vi "Restarts by Flow Sandbox Original.vi"() -> ()   [LabVIEW 2013]
uses:
  Type Defs/CAN Mode.ctl
  Type Defs/Controller Names.ctl
  Type Defs/Controller List.ctl
  <vilib>/FPGAPlugInAG/sbRIO-9626/niLvFpga_Open_sbRIO-9626.vi
  <vilib>/rvi/interface/common/dynamic/niFpgaDynamicAddResources.vi
  <vilib>/rvi/interface/common/niFpgaWaitOnOcc.vi
  <vilib>/Utility/error.llb/Error Cluster From Error Code.vi
  <vilib>/rvi/errors/niLvFpgaAdjustHostInterfaceError.vi
  <vilib>/FPGAPlugInAG/Dynamic/niLvFpga_Reset_Dynamic.vi
  <vilib>/FPGAPlugInAG/Dynamic/niLvFpga_Run_Dynamic.vi
  <vilib>/rvi/interface/nirviOpenFPGA/nirviOpenFPGA.xnode
  FPGA/bitfiles/RestartsbyFlowOriginal.lvbitx
  <vilib>/rvi/interface/nirviMethod/nirviMethod.xnode
  <vilib>/rvi/interface/nirviReadWriteControl/nirviReadWriteControl.xnode
  NiFpgaLv.dll
  <vilib>/rvi/interface/Simulation/niFpgaSimulationCallBeginRW.vi
  <vilib>/NI_Real-Time Target Support.lvlib
  <vilib>/FPGAPlugInAG/Dynamic/niLvFpga_ReadFifo_Dynamic.vi
  <vilib>/rvi/errors/niLvFpgaMergeErrorWithErrorCode.vi
  <vilib>/FPGAPlugInAG/Dynamic/niLvFpga_ConfigureFifo_Dynamic.vi
panel:
  out "Pressure":dbl
  out "DetPres Starts":u32
  out "Pressure Graph":dbl[][](graph)
  out "Reset Restarts 2":bool
  out "Negative Threshold":dbl
  out "Positive Threshold":dbl
  out "Armed":bool
  out "Flow":dbl
  out "Alt Flow Starts":u32
  out "Current":fxp<+/-,28,17>
  out "Current Graph":dbl[](graph)
  out "Init 2 Index":i32
  out "Commanded Starts":i16
  in  "Update Graph":bool=TRUE
  out "DetFlow Starts":u32
  in  "Position":i32=1
  in  "Seconds per Step":dbl=1.5 min=0.25 max=500.0 step=0.25
  out "Case":string
  in  "PreDataPts":i32=2000
  in  "Stop Init 2":bool
  out "Data Points":u32
  out "Current Step":i32
  in  "Reset Restarts":bool
  out "Flow Graph":dbl[](graph)
  in  "Profile":dbl[][](array[numeric])=[[1.25, 0.0, 0.0], [1.25, 650.0, 700.0]]
  in  "Run profile?":bool
  out "CFR 2":u64 format="%.0x"
  out "CFR2":u64 format="%.0x"
  in  "Pressure":dbl min=0.0 max=800.0 step=1.0 format="%#_13g"
  out "CPU Usage:":dbl=7.74131899555212 format="%.1f"
  in  "CAN CMD":dbl min=0.0 max=800.0 step=1.0
  # "cmd"
  # "pres"
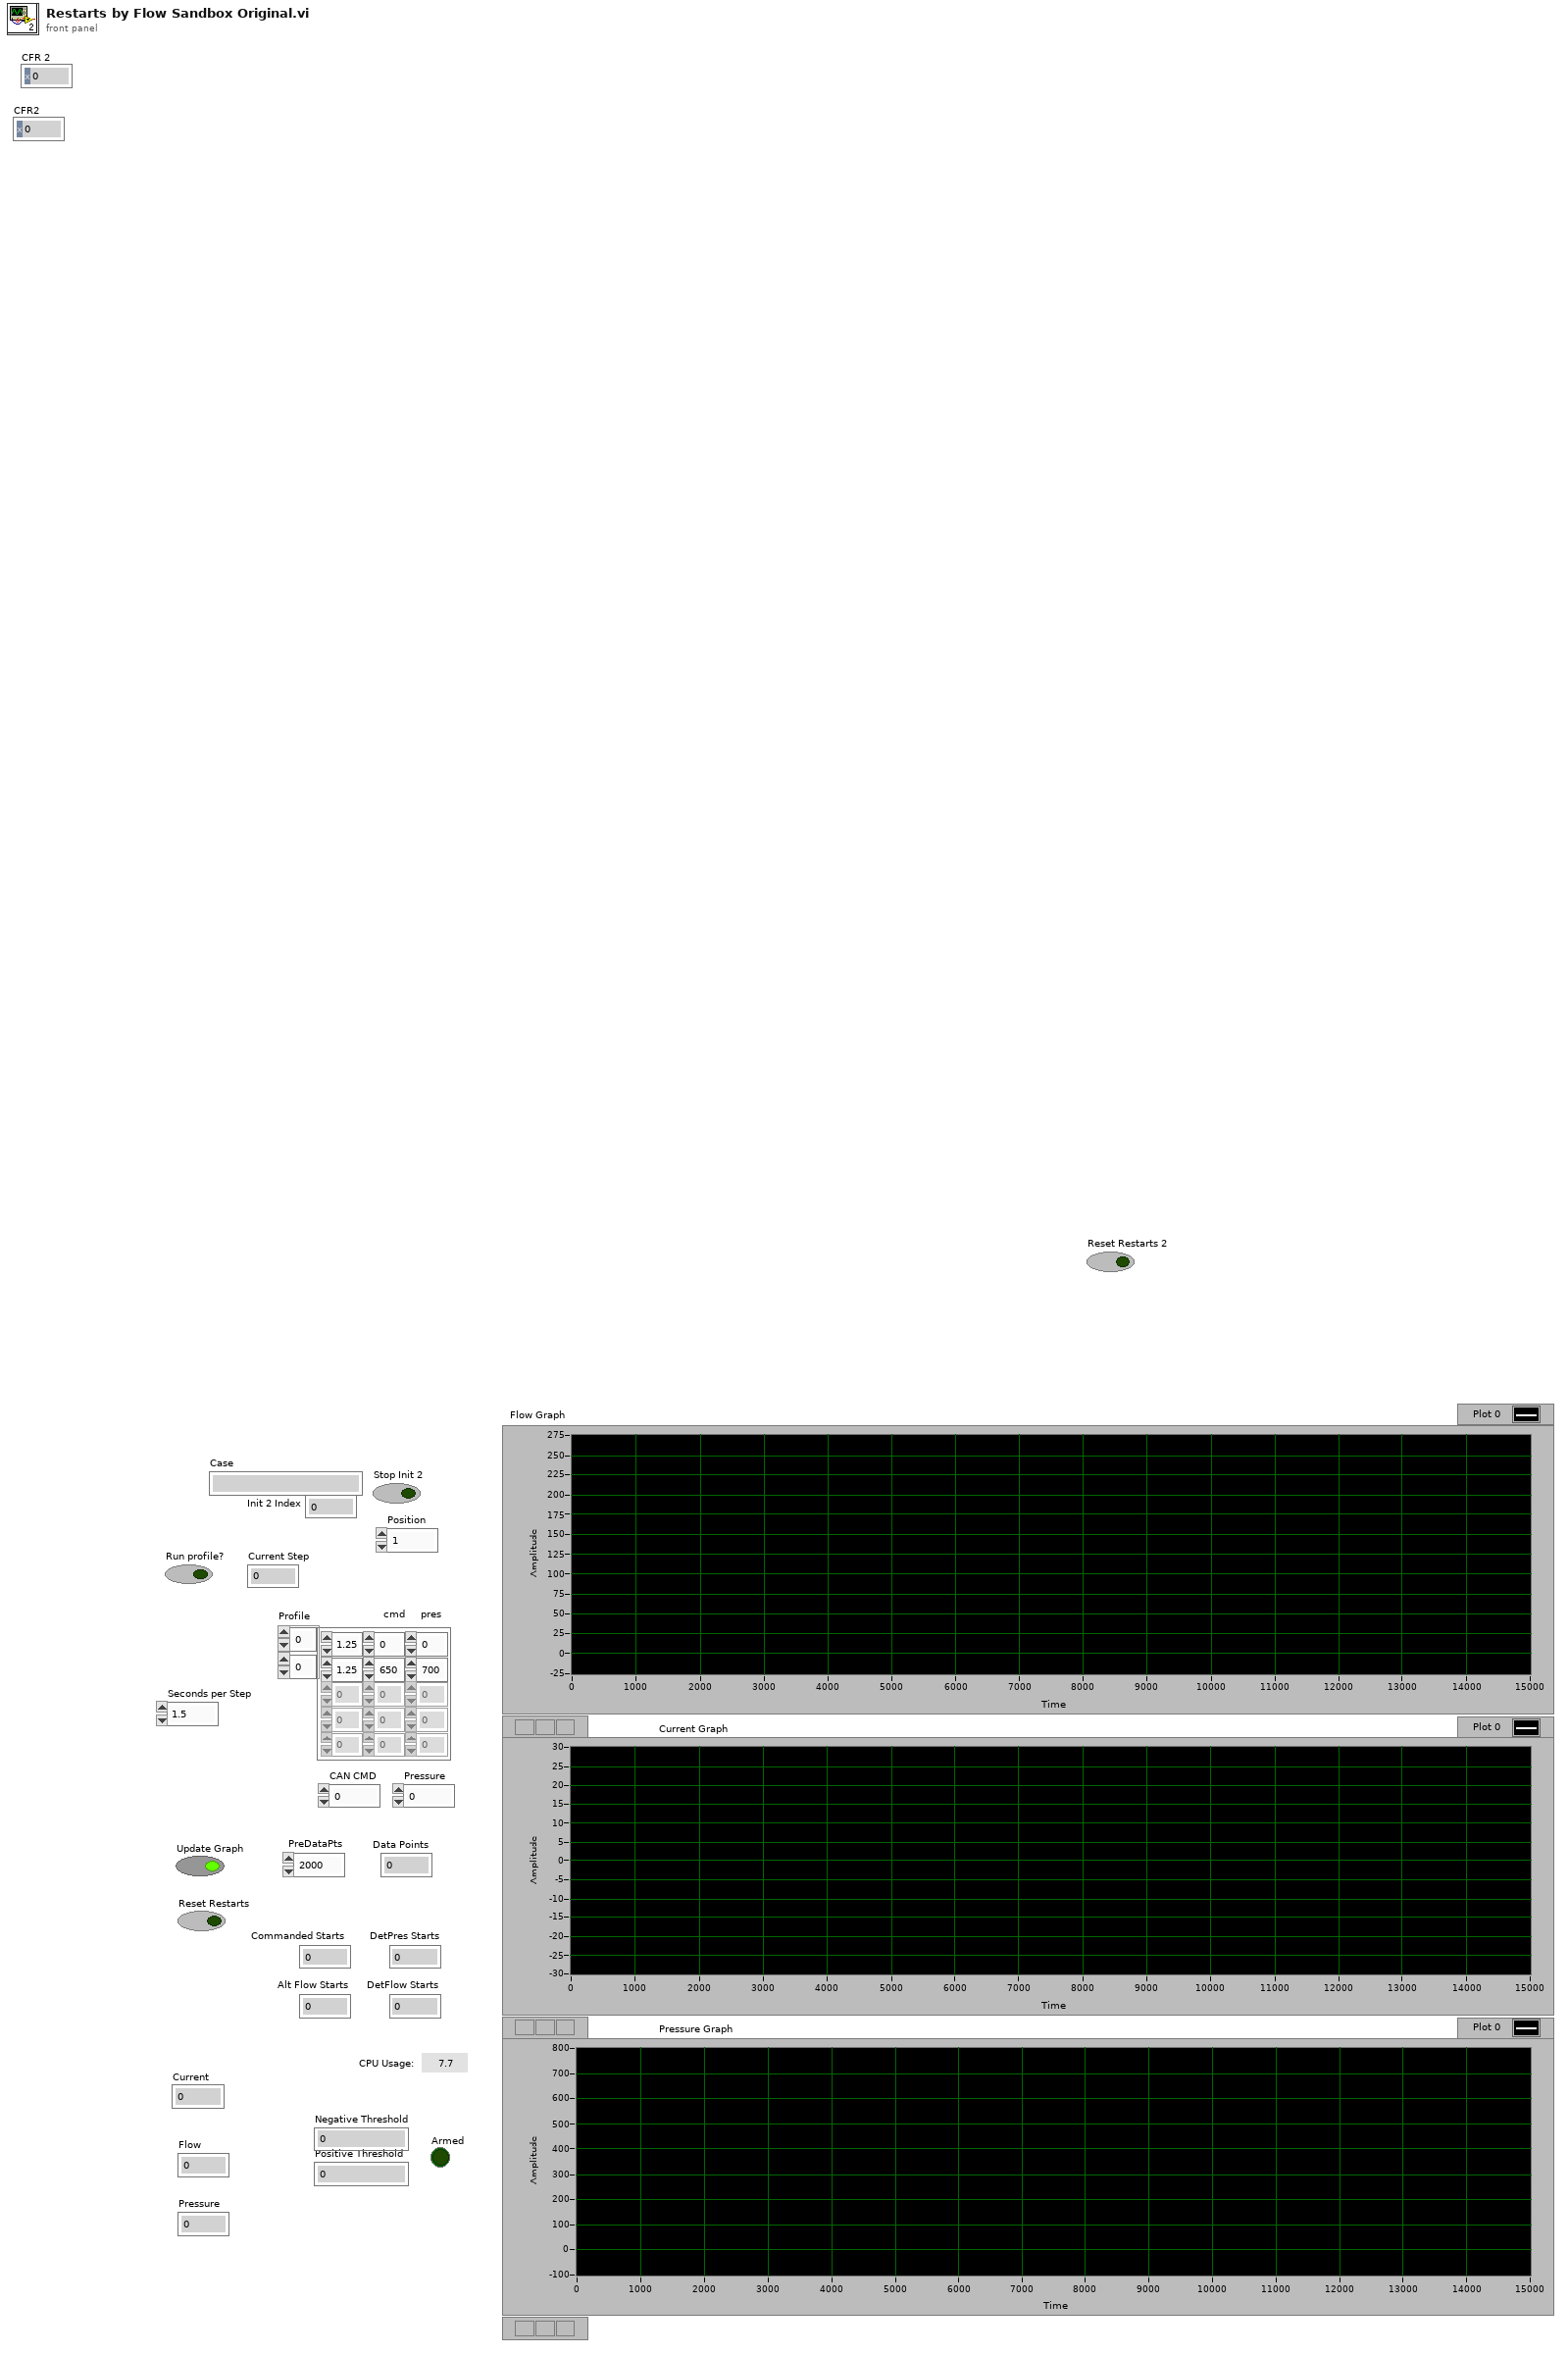
[diagram p1: front panel]
types:
  T1 = typedef "CAN Mode.ctl" = enum16{"Init", "Read", "Write", "Close"}
  T2 = typedef "Controller Names.ctl" = enum16{"Kuhnke", "Conti", "Helbako", "TI PWM", "PSA", "Hella Gas", "Hella Diesel", "8 Comm", "10 Comm", "8 Comm Hella", "10 Comm Hella", "8 Comm Omron", "10 Comm Omron", "8 Comm Nissan", "10 Comm Nissan"}
  T3 = typedef "Controller List.ctl" = cluster{"Controller Name":T2, "CommSeg":i32, "PWM?":bool, "Frequency":i32, "Low Command":dbl, "High Command":dbl, "Stop Command":dbl, "Command Step":dbl, "Solenoid Stop?":bool, "Controller?":bool}[]
  T4 = cluster{"Divide Value":u8, "Transfer Length (bits)":u8, "CS Asserted Polarity":bool, "Clock Polarity (CPOL)":bool, "Clock Phase (CPHA)":bool, "Lengthen MISO Setup":bool, "Direction Change Bit":u8, "MOSI Starts as Output":bool, "Tristatable MOSI":bool}
  T5 = cluster{"Controller Name":T2, "CommSeg":i32, "PWM?":bool, "Frequency":i32, "Low Command":dbl, "High Command":dbl, "Stop Command":dbl, "Command Step":dbl, "Solenoid Stop?":bool, "Controller?":bool}
  T6 = typedef "NI_Real-Time Target Support.lvlib/RT CPU Load.ctl" = cluster{"Total (%)":dbl, "Time Critical (%)":dbl, "Timed Structures (%)":dbl, "High (%)":dbl, "Above Normal (%)":dbl, "Normal (%)":dbl, "Background (%)":dbl, "Idle (%)":dbl, "ISR (%)":dbl}
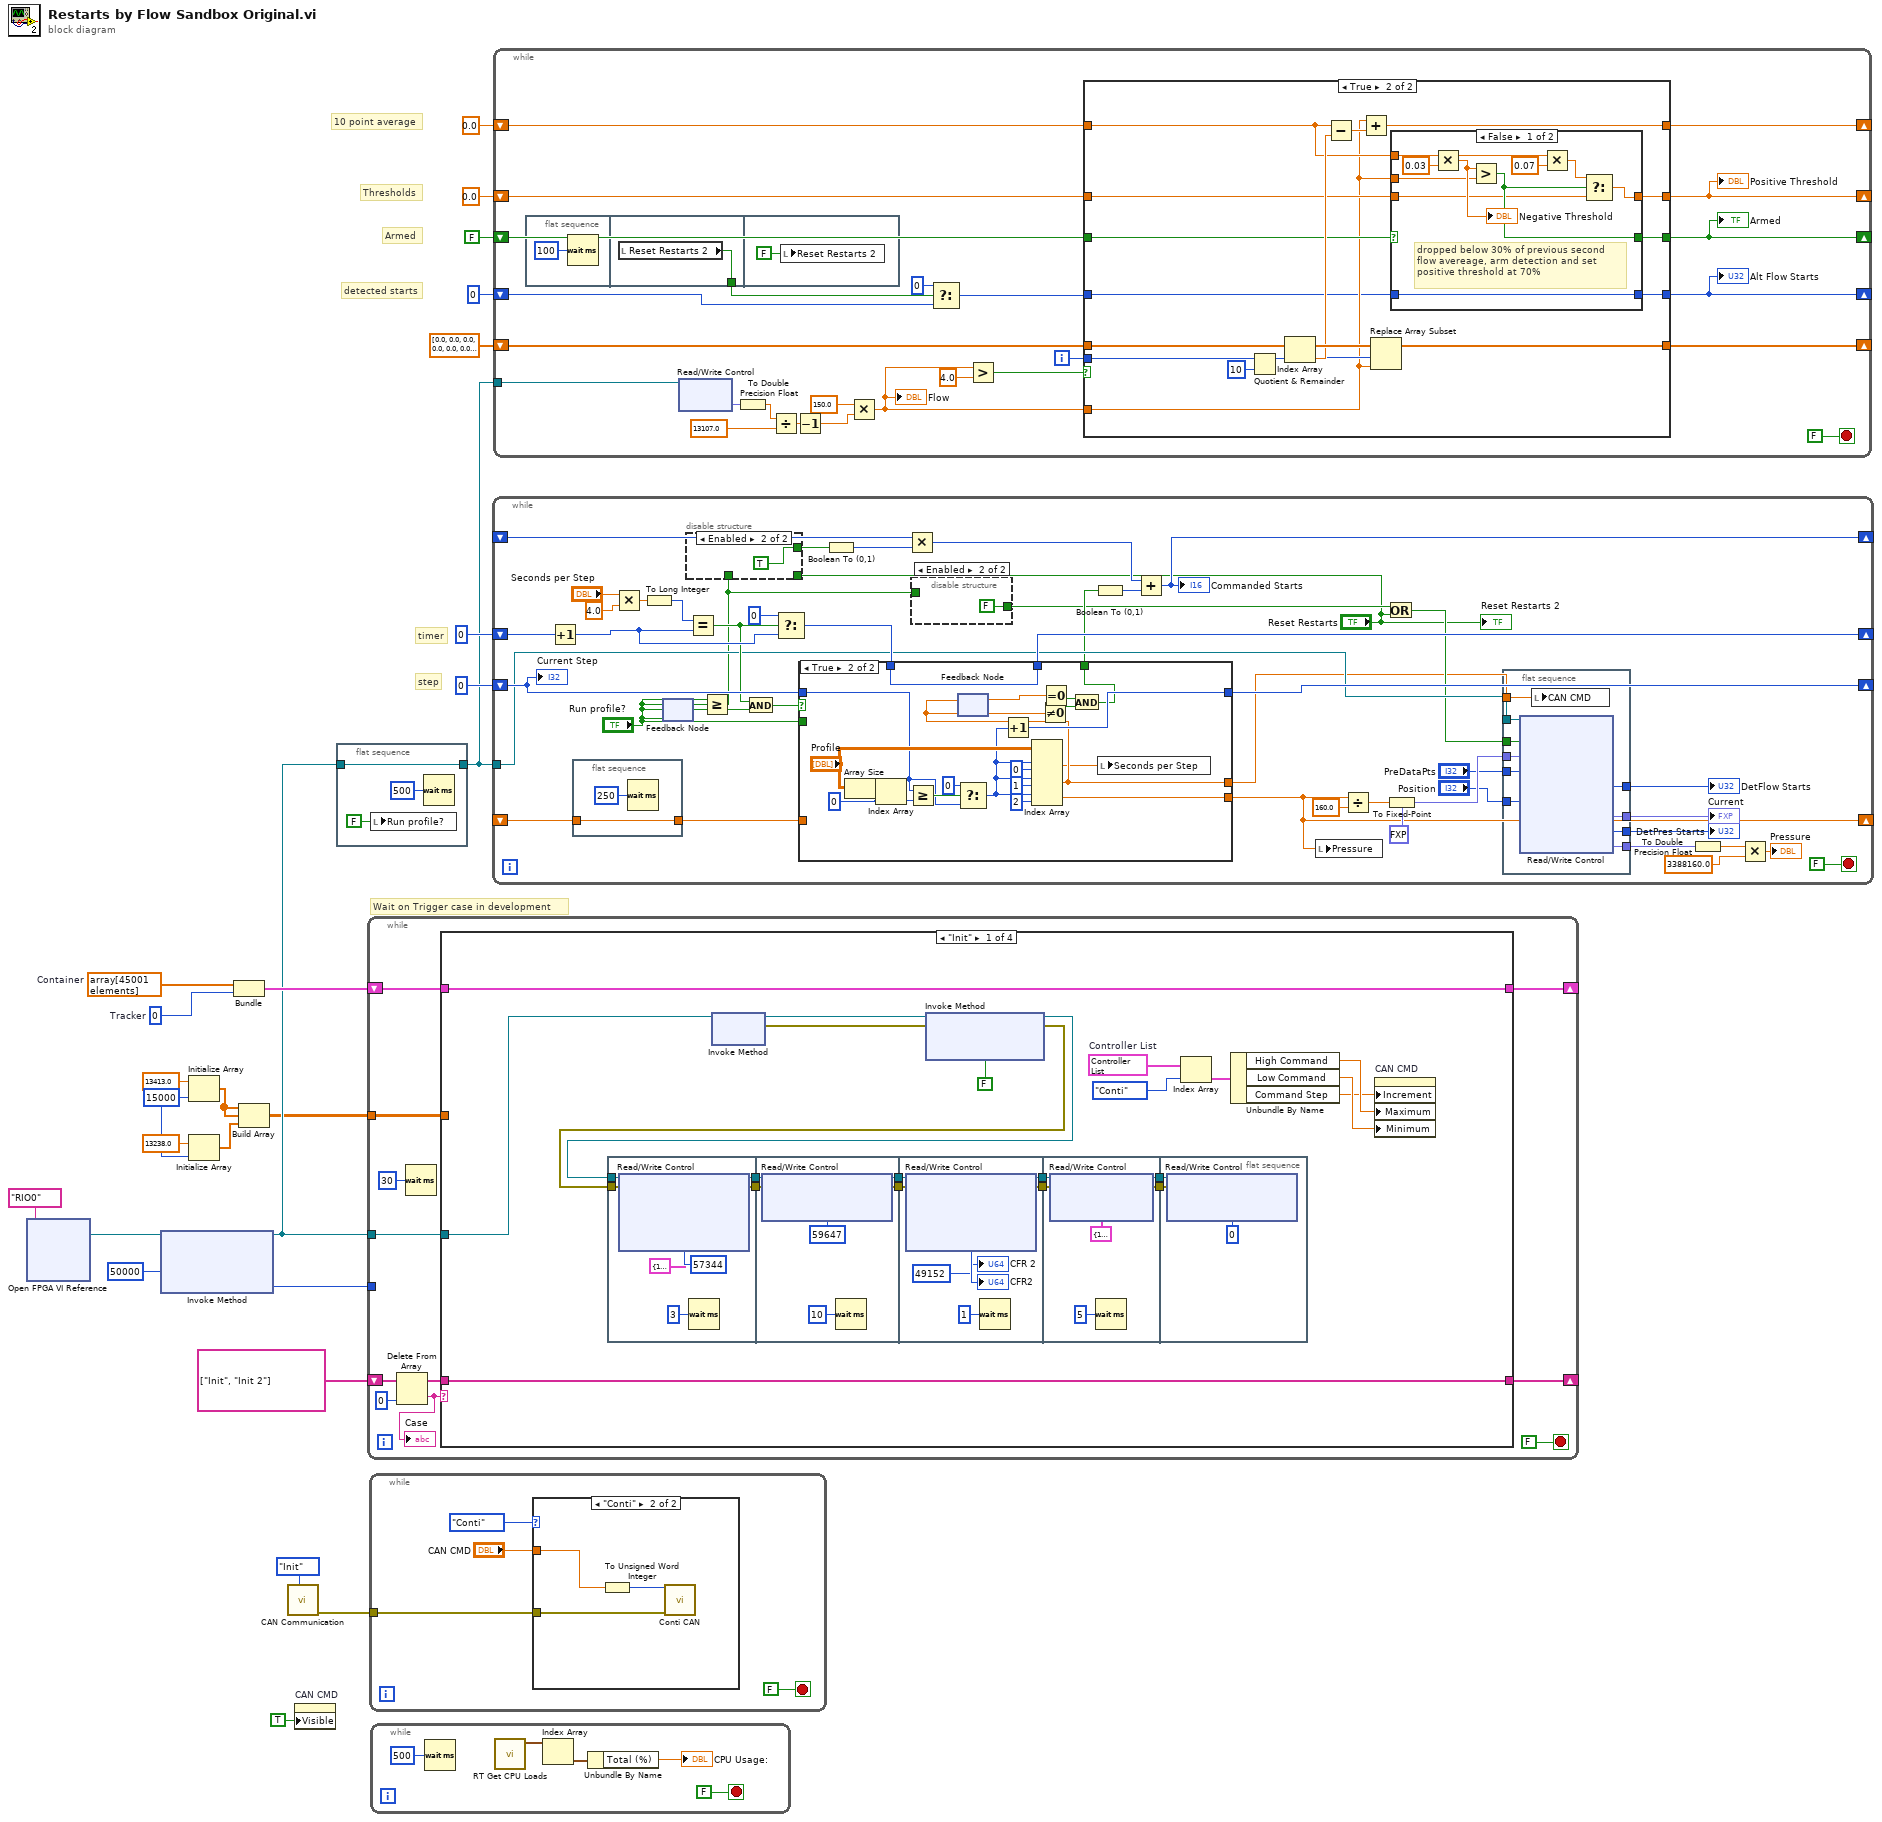
[diagram p0: block diagram]
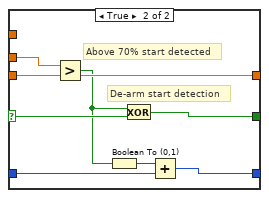
[diagram p3: hidden frame]
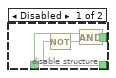
[diagram p4: hidden frame]
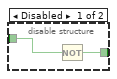
[diagram p5: hidden frame]
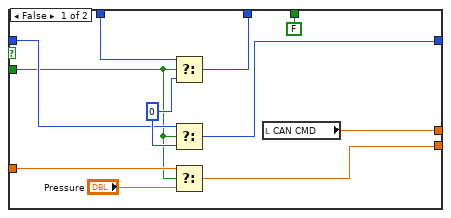
[diagram p6: hidden frame]
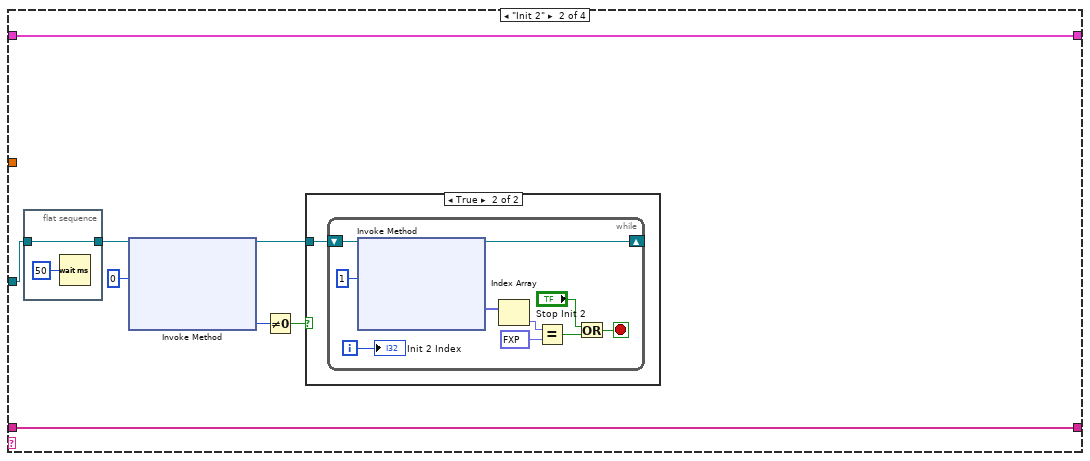
[diagram p7: hidden frame]
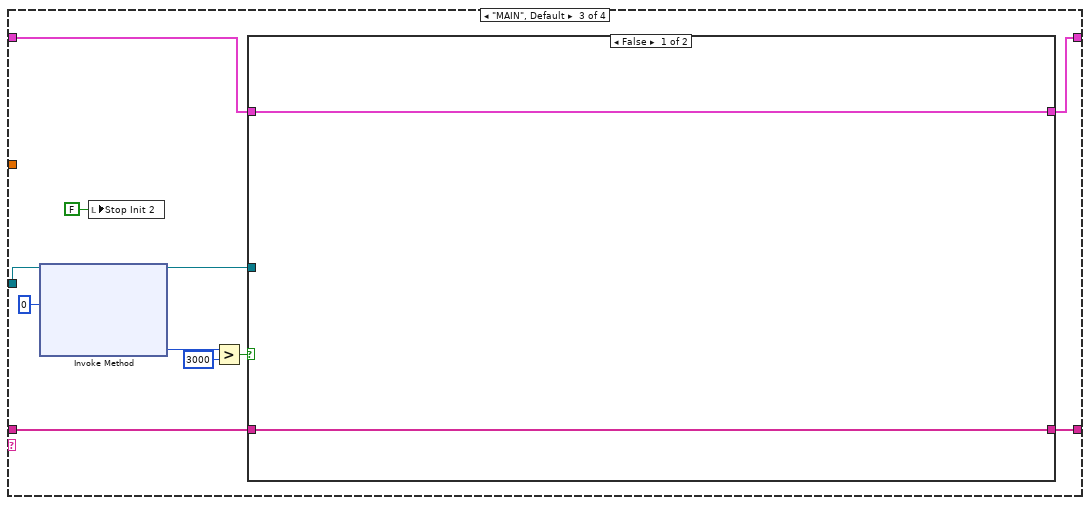
[diagram p9: hidden frame]
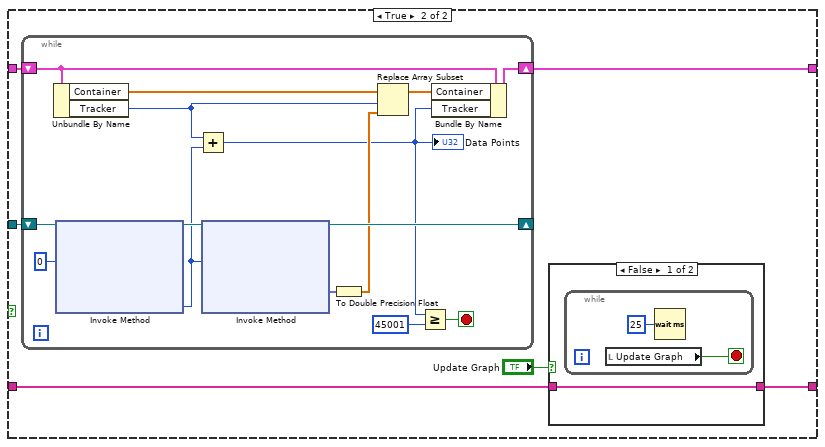
[diagram p10: hidden frame]
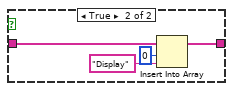
[diagram p11: hidden frame]
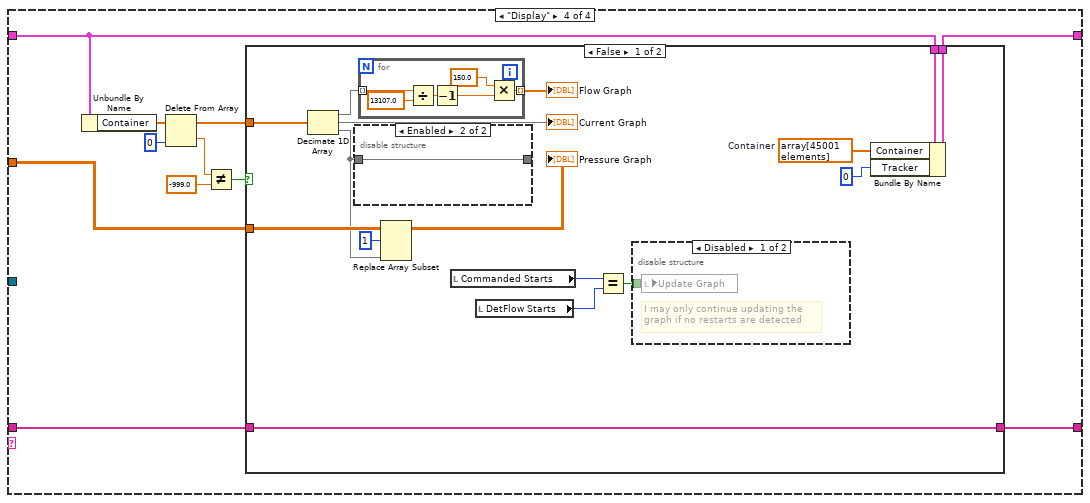
[diagram p12: hidden frame]
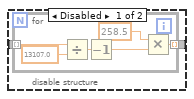
[diagram p13: hidden frame]
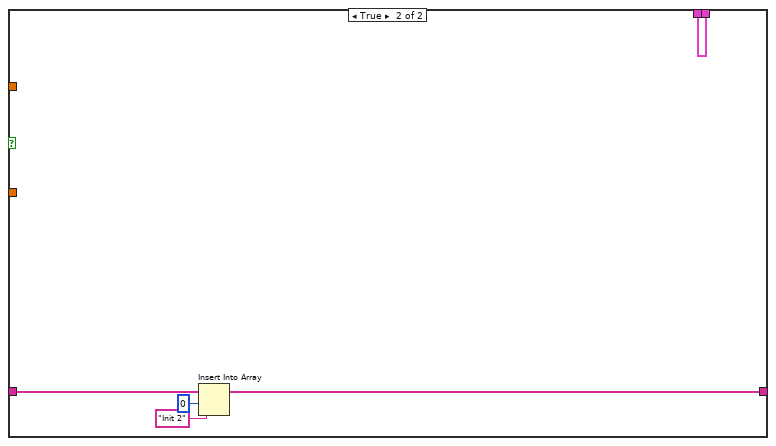
[diagram p15: hidden frame]
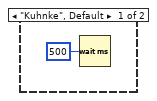
[diagram p16: hidden frame]
diagram:
  w6 = 15000 ("dimension size")
  w13 = u32 0  # Tracker
  w17 = dbl[] array[45001 elements]  # Container
  # "Armed"
  # "Thresholds"
  # "detected starts"
  # "10 point average"
  # "timer"
  # "step"
  # "Wait on Trigger case in development"
  n1 = xnode "Open FPGA VI Reference"("resource name"=tag "RIO0") -> ("FPGA VI Reference Out"=w19:refnum<k20>)  [unwired: 1 in, 1 out]
  n2 = xnode "Invoke Method"("FPGA VI Reference In"=w19, "Requested Depth"=u32 50000) -> ("FPGA VI Reference Out"=w16:refnum<k20>, "Actual Depth"=w18:u32)  [unwired: 1 in, 1 out]
  n3 = Initialize Array(13413.0 ("element"), w6) -> (w2:dbl[])
  n4 = Initialize Array(13238.0 ("element"), w6) -> (w3:dbl[])
  n5 = Bundle("Container"=w17, "Tracker"=w13) -> (w21:cluster{"Container":dbl[], "Tracker":u32})  [unwired: 1 in]
  n6 = Build Array(w2, w2, w3) -> (w1:dbl[][])
  n7 = call "CAN Communication.vi"("CAN Mode"=CAN_Mode."Init") -> ("Error OUT"=w23:errorcluster)  [unwired: 10 in]
  n8 = property on="CAN CMD" class="DigNum (strict)"("Visible"=TRUE) -> ()  [unwired: 2 in, 2 out]
  n9 = flat-sequence {
    tunnel: w16 -> [w29]
    tunnel: [w29] -> w11
    frame #0 {
      n10 = local write "Run profile?"(FALSE ("Run profile?")) -> ()
      n11 = Wait (ms)(milliseconds to wait=u32 500) -> ()  [unwired: 1 out]
    }
  }
  n12 = while {
    shift-right: [w37] -> _
    shift-left: string[] ["Init", "Init 2"] -> [w40]
    shift-right: [w34] -> _
    shift-left: w21 -> [w35]
    tunnel: w16 -> [w33]
    tunnel: w18 -> [_]
    tunnel: w1 -> [w30]
    stop <- FALSE stop-if-true
    n13 = Delete From Array(array=w40, index=0) -> (deleted portion=w31:string, array with subset deleted=w38:string[])  [unwired: 1 in]
    "Case" <- w31
    n14 = Wait (ms)(milliseconds to wait=u32 30) -> ()  [unwired: 1 out]
    n15 = case shown="\"Init\"" w31 {
      tunnel: w38 -> [w62 w99 w120 w160]
      tunnel: [w62 w99 w119 w159] -> w37
      tunnel: w35 -> [w61 w100 w117 w157]
      tunnel: [w61 w100 w116 w156] -> w34
      tunnel: w33 -> [w60 w94 w124 _]
      tunnel: w30 -> [_ _ _ w155]
      frame "Init" {
        w42 = T3 [{"Controller Name"=enum."Kuhnke", "CommSeg"=2, "PWM?"=TRUE, "Frequency"=100, "Low Command"=10.0, "High Command"=100.0, "Stop Command"=10.0, "Command Step"=0.1, "Solenoid Stop?"=FALSE, "Controller?"=FALSE}, {"Controller Name"=enum."Conti", "CommSeg"=2, "PWM?"=FALSE, "Frequency"=100, "Low Command"=0.0, "High Command"=800.0, "Stop Command"=0.0, "Command Step"=1.0, "Solenoid Stop?"=FALSE, "Controller?"=FALSE}, {"Controller Name"=enum."Helbako", "CommSeg"=2, "PWM?"=FALSE, "Frequency"=100, "Low Command"=0.0, "High Command"=100.0, "Stop Command"=0.0, "Command Step"=0.1, "Solenoid Stop?"=FALSE, "Controller?"=FALSE}, {"Controller Name"=enum."TI PWM", "CommSeg"=2, "PWM?"=TRUE, "Frequency"=100, "Low Command"=0.0, "High Command"=100.0, "Stop Command"=0.0, "Command Step"=0.1, "Solenoid Stop?"=FALSE, "Controller?"=FALSE}, {"Controller Name"=enum."PSA", "CommSeg"=2, "PWM?"=TRUE, "Frequency"=100, "Low Command"=5.0, "High Command"=95.0, "Stop Command"=5.0, "Command Step"=0.1, "Solenoid Stop?"=FALSE, "Controller?"=FALSE}, {"Controller Name"=enum."Hella Gas", "CommSeg"=2, "PWM?"=FALSE, "Frequency"=100, "Low Command"=0.0, "High Command"=800.0, "Stop Command"=0.0, "Command Step"=1.0, "Solenoid Stop?"=TRUE, "Controller?"=FALSE}, {"Controller Name"=enum."Hella Diesel", "CommSeg"=2, "PWM?"=FALSE, "Frequency"=100, "Low Command"=370.0, "High Command"=461.0, "Stop Command"=370.0, "Command Step"=1.0, "Solenoid Stop?"=TRUE, "Controller?"=FALSE}, {"Controller Name"=enum."8 Comm", "CommSeg"=8, "PWM?"=FALSE, "Frequency"=100, "Low Command"=0.0, "High Command"=1.0, "Stop Command"=0.0, "Command Step"=1.0, "Solenoid Stop?"=FALSE, "Controller?"=FALSE}, {"Controller Name"=enum."10 Comm", "CommSeg"=10, "PWM?"=FALSE, "Frequency"=100, "Low Command"=0.0, "High Command"=1.0, "Stop Command"=0.0, "Command Step"=1.0, "Solenoid Stop?"=FALSE, "Controller?"=FALSE}, {"Controller Name"=enum."8 Comm Hella", "CommSeg"=8, "PWM?"=TRUE, "Frequency"=150, "Low Command"=0.0, "High Command"=50.0, "Stop Command"=80.0, "Command Step"=0.1, "Solenoid Stop?"=FALSE, "Controller?"=FALSE}, {"Controller Name"=enum."10 Comm Hella", "CommSeg"=10, "PWM?"=TRUE, "Frequency"=150, "Low Command"=0.0, "High Command"=50.0, "Stop Command"=80.0, "Command Step"=0.1, "Solenoid Stop?"=FALSE, "Controller?"=FALSE}, {"Controller Name"=enum."8 Comm Omron", "CommSeg"=8, "PWM?"=TRUE, "Frequency"=150, "Low Command"=5.0, "High Command"=50.0, "Stop Command"=75.0, "Command Step"=0.1, "Solenoid Stop?"=FALSE, "Controller?"=FALSE}, {"Controller Name"=enum."10 Comm Omron", "CommSeg"=10, "PWM?"=TRUE, "Frequency"=150, "Low Command"=5.0, "High Command"=50.0, "Stop Command"=75.0, "Command Step"=0.1, "Solenoid Stop?"=FALSE, "Controller?"=FALSE}, {"Controller Name"=enum."8 Comm Nissan", "CommSeg"=8, "PWM?"=TRUE, "Frequency"=10, "Low Command"=50.0, "High Command"=90.0, "Stop Command"=50.0, "Command Step"=0.1, "Solenoid Stop?"=TRUE, "Controller?"=FALSE}, {"Controller Name"=enum."10 Comm Nissan", "CommSeg"=10, "PWM?"=TRUE, "Frequency"=10, "Low Command"=50.0, "High Command"=90.0, "Stop Command"=50.0, "Command Step"=0.1, "Solenoid Stop?"=TRUE, "Controller?"=FALSE}]  # Controller List
        n16 = flat-sequence {
          tunnel: w46 -> [w68]
          tunnel: w45 -> [w66]
          tunnel: [w69] -> w54
          tunnel: [w67] -> w53
          tunnel: w54 -> [w74]
          tunnel: w53 -> [w73]
          tunnel: [w72] -> w52
          tunnel: [w71] -> w51
          tunnel: w52 -> [w80]
          tunnel: w51 -> [w79]
          tunnel: [w78] -> w50
          tunnel: [w77] -> w49
          tunnel: w50 -> [w88]
          tunnel: w49 -> [w87]
          tunnel: [w85] -> w48
          tunnel: [w84] -> w47
          tunnel: w48 -> [w91]
          tunnel: w47 -> [w90]
          frame #0 {
            w64 = T4 {"Divide Value"=1, "Transfer Length (bits)"=16, "CS Asserted Polarity"=FALSE, "Clock Polarity (CPOL)"=TRUE, "Clock Phase (CPHA)"=FALSE, "Lengthen MISO Setup"=FALSE, "Direction Change Bit"=0, "MOSI Starts as Output"=FALSE, "Tristatable MOSI"=FALSE} ("Master Settings")
            w65 = u64 57344 ("data to write")
            n17 = xnode "Read/Write Control"("FPGA VI Reference In"=w68, "error in"=w66, "AI16-23 Settings"=w64, "AI16-23 Data to Write"=w65, "AI24-31 Settings"=w64, "AI24-31 Data to Write"=w65) -> ("FPGA VI Reference Out"=w69:refnum<k20>, "error out"=w67:errorcluster)
            n18 = Wait (ms)(milliseconds to wait=u32 3) -> ()  [unwired: 1 out]
          }
          frame #1 {
            w75 = u64 59647 ("data to write")
            n19 = xnode "Read/Write Control"("FPGA VI Reference In"=w74, "error in"=w73, "AI16-23 Data to Write"=w75, "AI24-31 Data to Write"=w75) -> ("FPGA VI Reference Out"=w72:refnum<k20>, "error out"=w71:errorcluster)
            n20 = Wait (ms)(milliseconds to wait=u32 10) -> ()  [unwired: 1 out]
          }
          frame #2 {
            n21 = xnode "Read/Write Control"("FPGA VI Reference In"=w80, "error in"=w79, "AI24-31 Data to Write"=u64 49152 ("data to write")) -> ("FPGA VI Reference Out"=w78:refnum<k20>, "error out"=w77:errorcluster, "Read Data"=→"CFR 2":u64, "Read Data 2"=→"CFR2":u64)  [unwired: 1 in]
            n22 = Wait (ms)(milliseconds to wait=u32 1) -> ()  [unwired: 1 out]
          }
          frame #3 {
            w89 = T4 {"Divide Value"=1, "Transfer Length (bits)"=19, "CS Asserted Polarity"=FALSE, "Clock Polarity (CPOL)"=TRUE, "Clock Phase (CPHA)"=FALSE, "Lengthen MISO Setup"=FALSE, "Direction Change Bit"=0, "MOSI Starts as Output"=FALSE, "Tristatable MOSI"=FALSE} ("Master Settings")
            n23 = xnode "Read/Write Control"("FPGA VI Reference In"=w88, "error in"=w87, "AI16-23 Settings"=w89, "AI24-31 Settings"=w89) -> ("FPGA VI Reference Out"=w85:refnum<k20>, "error out"=w84:errorcluster)
            n24 = Wait (ms)(milliseconds to wait=u32 5) -> ()  [unwired: 1 out]
          }
          frame #4 {
            w92 = u64 0 ("AI16-23 Data to Write")
            n25 = xnode "Read/Write Control"("FPGA VI Reference In"=w91, "error in"=w90, "AI16-23 Data to Write"=w92, "AI24-31 Data to Write"=w92) -> ()  [unwired: 2 out]
          }
        }
        n26 = xnode "Invoke Method"("FPGA VI Reference In"=w60) -> ("FPGA VI Reference Out"=w44:refnum<k20>, "error out"=w43:errorcluster)  [unwired: 1 in]
        n27 = xnode "Invoke Method"("FPGA VI Reference In"=w44, "error in"=w43, "Wait Until Done (F)"=FALSE) -> ("FPGA VI Reference Out"=w46:refnum<k20>, "error out"=w45:errorcluster)
        n28 = Index Array(array=w42, index=Controller_Names."Conti" ("Controller Type:")) -> (element=w56:T5)
        n29 = Unbundle By Name(w56) -> ("High Command"=w59:dbl, "Low Command"=w58:dbl, "Command Step"=w57:dbl)
        n30 = property on="CAN CMD" class="DigNum (strict)"("Increment"=w57, "Maximum"=w59, "Minimum"=w58) -> ()  [unwired: 2 in, 2 out]
      }
      frame "Init 2" {
        n31 = flat-sequence {
          tunnel: w94 -> [w101]
          tunnel: [w101] -> w93
          frame #0 {
            n32 = Wait (ms)(milliseconds to wait=u32 50) -> ()  [unwired: 1 out]
          }
        }
        n33 = xnode "Invoke Method"("FPGA VI Reference In"=w93, "Number of Elements"=u32 0) -> ("FPGA VI Reference Out"=w95:refnum<k20>, "Elements Remaining"=w97:u32)  [unwired: 2 in, 2 out]
        n34 = Not Equal To 0?(x=w97) -> (x != 0?=w96:bool)
        n35 = case shown="True" w96 {
          tunnel: w95 -> [_ w103]
          frame False {
          }
          frame True {
            n36 = while {
              shift-right: [w112] -> _
              shift-left: w103 -> [w113]
              i -> [w106]
              stop <- w107 stop-if-true
              n37 = xnode "Invoke Method"("FPGA VI Reference In"=w113, "Number of Elements"=u32 1) -> ("FPGA VI Reference Out"=w112:refnum<k20>, "Data"=w110:fxp<+/-,28,17>[])  [unwired: 2 in, 2 out]
              n38 = Index Array(array=w110) -> (element=w109:fxp<+/-,28,17>)  [unwired: 1 in]
              n39 = Equal?(x=w109, y=fxp<+/-,28,17> -999.0) -> (x = y?=w104:bool)
              n40 = Or(x="Stop Init 2", y=w104) -> (x .or. y?=w107:bool)
              "Init 2 Index" <- w106
            }
          }
        }
      }
      frame "MAIN", Default {
        n41 = xnode "Invoke Method"("FPGA VI Reference In"=w124, "Number of Elements"=u32 0) -> ("FPGA VI Reference Out"=w115:refnum<k20>, "Elements Remaining"=w122:u32)  [unwired: 2 in, 2 out]
        n42 = local write "Stop Init 2"(FALSE ("Stop Init 2")) -> ()
        n43 = Greater?(x=w122, y=u32 3000) -> (0:w118:bool)
        n44 = case shown="False" w118 {
          tunnel: w120 -> [w126 w129]
          tunnel: [w126 w128] -> w119
          tunnel: w117 -> [w125 w132]
          tunnel: [w125 w131] -> w116
          tunnel: w115 -> [_ w130]
          frame False {
          }
          frame True {
            n45 = while {
              shift-right: [w153] -> w131
              shift-left: w132 -> [w154]
              shift-right: [w149] -> _
              shift-left: w130 -> [w152]
              stop <- w140 stop-if-true
              n46 = Unbundle By Name(w154) -> ("Container"=w148:dbl[], "Tracker"=w144:u32)
              n47 = xnode "Invoke Method"("FPGA VI Reference In"=w152, "Number of Elements"=u32 0) -> ("FPGA VI Reference Out"=w150:refnum<k20>, "Elements Remaining"=w143:u32)  [unwired: 2 in, 2 out]
              n48 = Add(x=w144, y=w143) -> (x+y=w142:u32)
              "Data Points" <- w142
              n49 = xnode "Invoke Method"("FPGA VI Reference In"=w150, "Number of Elements"=w143) -> ("FPGA VI Reference Out"=w149:refnum<k20>, "Data"=w147:fxp<+/-,28,17>[])  [unwired: 2 in, 2 out]
              n50 = To Double Precision Float(number=w147) -> (double precision float=w145:dbl[])
              n51 = Replace Array Subset(array=w148, new element=w145, index=w144) -> (w146:dbl[])
              n52 = Greater Or Equal?(x=w142, y=u32 45001) -> (x >= y?=w140:bool)
              n53 = Bundle By Name(cluster=w154, "Container"=w146, "Tracker"=w142) -> (w153:cluster{"Container":dbl[], "Tracker":u32})
            }
            n54 = case shown="False" "Update Graph" {
              tunnel: w129 -> [w133 w137]
              tunnel: [w133 w136] -> w128
              frame False {
                n55 = while {
                  stop <- w135 stop-if-true
                  n56 = local read "Update Graph"() -> (w135:bool)
                  n57 = Wait (ms)(milliseconds to wait=u32 25) -> ()  [unwired: 1 out]
                }
              }
              frame True {
                n58 = Insert Into Array(array=w137, index=0, new element="Display" ("new element/subarray")) -> (w136:string[])
              }
            }
          }
        }
      }
      frame "Display" {
        n59 = Unbundle By Name(w157) -> ("Container"=w165:dbl[])
        n60 = Delete From Array(array=w165, index=0) -> (deleted portion=w163:dbl, array with subset deleted=w158:dbl[])  [unwired: 1 in]
        n61 = Not Equal?(x=w163, y=-999.0) -> (x != y?=w161:bool)
        n62 = case shown="False" w161 {
          tunnel: w160 -> [w181 w202]
          tunnel: [w181 w201] -> w159
          tunnel: w158 -> [w172 _]
          tunnel: w157 -> [w171 w198]
          tunnel: [w170 w198] -> w156
          tunnel: w155 -> [w169 _]
          frame False {
            w177 = dbl[] array[45001 elements]  # Container
            n63 = Decimate 1D Array(w172) -> (w179:dbl[], →"Current Graph":dbl[], w168:dbl[])
            n64 = disable-structure shown="Enabled" {
              disable-tunnel: w168 -> [w183 w190]
              disable-tunnel: [w182 w190] -> _
              frame Disabled {
                n65 = for {
                  tunnel: w183 -> [w185] mode=indexing
                  tunnel: [w184] -> w182 mode=indexing
                  n66 = Divide(x=w185, y=13107.0) -> (x/y=w187:dbl)
                  n67 = Decrement(x=w187) -> (x-1=w188:dbl)
                  n68 = Multiply(x=258.5, y=w188) -> (x*y=w184:dbl)
                }
              }
              frame Enabled {
              }
            }
            n69 = for {
              tunnel: w179 -> [w193] mode=indexing
              tunnel: [w192] -> w180 mode=indexing
              n70 = Divide(x=w193, y=13107.0) -> (x/y=w195:dbl)
              n71 = Decrement(x=w195) -> (x-1=w196:dbl)
              n72 = Multiply(x=150.0, y=w196) -> (x*y=w192:dbl)
            }
            "Flow Graph" <- w180
            n73 = Replace Array Subset(array=w169, new element=w168, index (row)=1) -> (→"Pressure Graph":dbl[][])  [unwired: 1 in]
            n74 = local read "Commanded Starts"() -> (w175:i16)
            n75 = local read "DetFlow Starts"() -> (w176:u32)
            n76 = Equal?(x=w175, y=w176) -> (x = y?=w174:bool)
            n77 = disable-structure shown="Disabled" {
              disable-tunnel: w174 -> [w191 _]
              frame Disabled {
                # "I may only continue updating the\ngraph if no restarts are detected"
                n78 = local write "Update Graph"(w191) -> ()
              }
              frame Enabled {
              }
            }
            n79 = Bundle By Name(cluster=w171, "Container"=w177, "Tracker"=u32 0 ("DataPoints")) -> (w170:cluster{"Container":dbl[], "Tracker":u32})
          }
          frame True {
            n80 = Insert Into Array(array=w202, index=0, new element="Init 2" ("new element/subarray")) -> (w201:string[])
          }
        }
      }
    }
  }
  n81 = while {
    tunnel: w23 -> [w205]
    stop <- FALSE stop-if-true
    n82 = case shown="\"Conti\"" Controller_Names."Conti" ("Controller Type:") {
      tunnel: w205 -> [_ w210]
      tunnel: "CAN CMD" -> [_ w209]
      frame "Kuhnke", Default {
        n83 = Wait (ms)(milliseconds to wait=u32 500) -> ()  [unwired: 1 out]
      }
      frame "Conti" {
        n84 = To Unsigned Word Integer(number=w209) -> (unsigned 16bit integer=w208:u16)
        n85 = call "Conti CAN.vi"("Error IN"=w210, "CMD"=w208) -> ()  [unwired: 9 in, 1 out]
      }
    }
  }
  n86 = while {
    stop <- FALSE stop-if-true
    n87 = Wait (ms)(milliseconds to wait=u32 500) -> ()  [unwired: 1 out]
    n88 = call <vilib>:"RT Get CPU Loads.vi"() -> ("CPU loads"=w212:T6[])  [unwired: 10 in, 1 out]
    n89 = Index Array(array=w212) -> (element=w213:T6)  [unwired: 1 in]
    n90 = Unbundle By Name(w213) -> ("Total (%)"=→"CPU Usage:":dbl)
  }
  n91 = while {
    tunnel: w11 -> [w241]
    shift-right: [w254] -> _
    shift-left: 0 ("disabled index (col)") -> [w255]
    shift-right: [w249] -> _
    shift-left: 0 ("disabled index (col)") -> [w253]
    shift-right: [w225] -> _
    shift-left: _ -> [w247]
    shift-right: [w236] -> _
    shift-left: _ -> [w234]
    stop <- FALSE stop-if-true
    n92 = Increment(x=w253) -> (x+1=w248:i32)
    n93 = flat-sequence {
      tunnel: w247 -> [w280]
      tunnel: [w280] -> w246
      frame #0 {
        n94 = Wait (ms)(milliseconds to wait=u32 250) -> ()  [unwired: 1 out]
      }
    }
    n95 = Multiply(x="Seconds per Step", y=4.0) -> (x*y=w230:dbl)
    n96 = To Long Integer(number=w230) -> (32bit integer=w229:i32)
    n97 = feedback #1("Run profile?") -> (w231:bool)
    n98 = feedback-in #1("Run profile?") -> ()
    n99 = Equal?(x=w229, y=w248) -> (x = y?=w245:bool)
    n100 = Greater Or Equal?(x="Run profile?", y=w231) -> (x >= y?=w224:bool)
    n101 = disable-structure shown="Enabled" {
      disable-tunnel: w224 -> [w264 _]
      disable-tunnel: [w263 TRUE] -> w223
      disable-tunnel: "Reset Restarts" -> [w262 _]
      frame Disabled {
        n102 = Not(x=w262) -> (.not. x?=w261:bool)
        n103 = And(x=w264, y=w261) -> (x .and. y?=w263:bool)
      }
      frame Enabled {
      }
    }
    n104 = And(x=w245, y="Run profile?") -> (x .and. y?=w252:bool)
    n105 = Select(t=0, s=w245, f=w248) -> (s? t:f=w250:i32)
    n106 = case shown="True" w252 {
      tunnel: [w287 w309] -> w225
      tunnel: w255 -> [w285 w302]
      tunnel: [w283 w300] -> w254
      tunnel: w250 -> [w291 w301]
      tunnel: [w290 w301] -> w249
      tunnel: "Run profile?" -> [w284 _]
      tunnel: w246 -> [w289 _]
      tunnel: [FALSE w299] -> w238
      tunnel: [w281 w295] -> w226
      frame False {
        w286 = 0 ("disabled index (col)")
        n107 = Select(t=w291, s=w284, f=w286) -> (s? t:f=w290:i32)
        n108 = Select(t=w285, s=w284, f=w286) -> (s? t:f=w283:i32)
        n109 = Select(t=w289, s=w284, f="Pressure") -> (s? t:f=w287:dbl)
        n110 = local read "CAN CMD"() -> (w281:dbl)
      }
      frame True {
        n111 = Array Size(array="Profile") -> (size(s)=w307:i32[])
        n112 = Index Array(array=w307, index=0 ("disabled index (col)")) -> (element=w305:i32)
        n113 = Greater Or Equal?(x=w302, y=w305) -> (x >= y?=w304:bool)
        n114 = Select(t=0, s=w304, f=w302) -> (s? t:f=w294:i32)
        n115 = Increment(x=w294) -> (x+1=w300:i32)
        n116 = Index Array(array="Profile", index (row) #1=w294, index (col) #1=0 ("disabled index (col)"), index (row) #2=w294, index (col) #2=1 ("disabled index (col)"), index (row) #3=w294, index (col) #3=2 ("disabled index (col)")) -> (element #1=w292:dbl, element #2=w295:dbl, element #3=w309:dbl)
        n117 = feedback-in #2(w295) -> ()
        n118 = feedback #2(w295) -> (w296:dbl)
        n119 = Not Equal To 0?(x=w295) -> (x != 0?=w297:bool)
        n120 = Equal To 0?(x=w296) -> (x = 0?=w298:bool)
        n121 = And(x=w298, y=w297) -> (x .and. y?=w299:bool)
        n122 = local write "Seconds per Step"(w292) -> ()
      }
    }
    n123 = Boolean To (0,1)(Boolean=w223) -> (0, 1=w235:i16)
    n124 = Multiply(x=w234, y=w235) -> (x*y=w233:i16)
    n125 = disable-structure shown="Enabled" {
      disable-tunnel: [w267 FALSE] -> w228
      disable-tunnel: w224 -> [w266 _]
      frame Disabled {
        n126 = Not(x=w266) -> (.not. x?=w267:bool)
      }
      frame Enabled {
      }
    }
    n127 = Boolean To (0,1)(Boolean=w238) -> (0, 1=w237:i16)
    n128 = Add(x=w233, y=w237) -> (x+y=w236:i16)
    "Commanded Starts" <- w236
    n129 = local write "Pressure"(w225) -> ()
    n130 = Divide(x=w225, y=160.0) -> (x/y=w257:dbl)
    n131 = Or(x=w228, y="Reset Restarts") -> (x .or. y?=w227:bool)
    n132 = To Fixed-Point(fixed-point type=fxp<+/-,20,5> 0.0 ("AO0"), number=w257) -> (fixed-point=w256:fxp<+/-,20,5>)
    n133 = flat-sequence {
      tunnel: w256 -> [w278]
      tunnel: "PreDataPts" -> [w277]
      tunnel: w241 -> [w276]
      tunnel: "Position" -> [w275]
      tunnel: [w274] -> w239
      tunnel: w227 -> [w273]
      tunnel: w226 -> [w272]
      tunnel: [w271] -> w221
      tunnel: [w270] -> w220
      tunnel: [w269] -> w219
      frame #0 {
        n134 = xnode "Read/Write Control"("FPGA VI Reference In"=w276, "Reset Restarts"=w273, "AO0"=w278, "PreDataPts"=w277, "Position"=w275) -> ("DetFlow Starts"=w274:u32, "Current"=w271:fxp<+/-,28,17>, "DetPres Starts"=w270:u32, "Pressure"=w269:fxp<+/-,28,17>)  [unwired: 1 in, 2 out]
        n135 = local write "CAN CMD"(w272) -> ()
      }
    }
    n136 = To Double Precision Float(number=w219) -> (double precision float=w218:dbl)
    n137 = Multiply(x=w218, y=3388160.0) -> (x*y=→"Pressure":dbl)
    "Current Step" <- w255
    "DetFlow Starts" <- w239
    "Current" <- w221
    "Reset Restarts 2" <- "Reset Restarts"
    "DetPres Starts" <- w220
  }
  n138 = while {
    shift-right: [w334] -> _
    shift-left: dbl[] [0.0, 0.0, 0.0, 0.0, 0.0, 0.0, 0.0, 0.0, 0.0, 0.0] -> [w335]
    shift-right: [w331] -> _
    shift-left: 0.0 -> [w332]
    shift-right: [w320] -> _
    shift-left: u32 0 -> [w318]
    shift-right: [w328] -> _
    shift-left: 0.0 -> [w333]
    shift-right: [w329] -> _
    shift-left: FALSE -> [w330]
    tunnel: w11 -> [w327]
    i -> [w312]
    stop <- FALSE stop-if-true
    n139 = flat-sequence {
      tunnel: [w377] -> w319
      frame #0 {
        n140 = Wait (ms)(milliseconds to wait=u32 100) -> ()  [unwired: 1 out]
      }
      frame #1 {
        n141 = local read "Reset Restarts 2"() -> (w377:bool)
      }
      frame #2 {
        n142 = local write "Reset Restarts 2"(FALSE ("Reset Restarts 2")) -> ()
      }
    }
    n143 = xnode "Read/Write Control"("FPGA VI Reference In"=w327) -> ("Flow"=w326:fxp<+/-,28,17>)  [unwired: 1 in, 2 out]
    n144 = To Double Precision Float(number=w326) -> (double precision float=w325:dbl)
    n145 = Divide(x=w325, y=13107.0) -> (x/y=w323:dbl)
    n146 = Decrement(x=w323) -> (x-1=w322:dbl)
    n147 = Multiply(x=150.0, y=w322) -> (x*y=w315:dbl)
    "Flow" <- w315
    n148 = Select(t=u32 0, s=w319, f=w318) -> (s? t:f=w316:u32)
    n149 = Greater?(x=w315, y=4.0) -> (0:w313:bool)
    n150 = case shown="True" w313 {
      tunnel: w335 -> [w341 w356]
      tunnel: [w341 w355] -> w334
      tunnel: w333 -> [w338 w353]
      tunnel: w332 -> [w337 w352]
      tunnel: [w337 w351] -> w331
      tunnel: w330 -> [w339 w350]
      tunnel: [w339 w349] -> w329
      tunnel: [w338 w348] -> w328
      tunnel: w315 -> [_ w345]
      tunnel: [w340 w344] -> w320
      tunnel: w316 -> [w340 w343]
      tunnel: w312 -> [_ w342]
      frame False {
      }
      frame True {
        n151 = Quotient & Remainder(x=w342, y=10) -> (x-y*floor(x/y)=w346:i32)  [unwired: 1 out]
        n152 = Index Array(array=w356, index=w346) -> (element=w354:dbl)
        n153 = Subtract(x=w352, y=w354) -> (x-y=w347:dbl)
        n154 = Add(x=w345, y=w347) -> (x+y=w351:dbl)
        n155 = Replace Array Subset(array=w356, new element=w345, index=w346) -> (w355:dbl[])
        n156 = case shown="False" w350 {
          selector: w350 -> [_ w370]
          tunnel: w352 -> [w364 _]
          tunnel: w345 -> [w365 w375]
          tunnel: [w362 w368] -> w349
          tunnel: w353 -> [w360 w371]
          tunnel: [w359 w371] -> w348
          tunnel: w343 -> [w358 w373]
          tunnel: [w358 w372] -> w344
          frame False {
            # "dropped below 30% of previous second\nflow avereage, arm detection and set\npositive threshold at 70%"
            n157 = Multiply(x=w364, y=0.03) -> (x*y=w366:dbl)
            "Negative Threshold" <- w366
            n158 = Greater?(x=w366, y=w365) -> (0:w362:bool)
            n159 = Multiply(x=w364, y=0.07) -> (x*y=w361:dbl)
            n160 = Select(t=w361, s=w362, f=w360) -> (s? t:f=w359:dbl)
          }
          frame True {
            # "De-arm start detection"
            # "Above 70% start detected"
            n161 = Greater?(x=w375, y=w371) -> (0:w369:bool)
            n162 = Boolean To (0,1)(Boolean=w369) -> (0, 1=w374:i16)
            n163 = Exclusive Or(1:w370, 2:w369) -> (0:w368:bool)
            n164 = Add(x=w374, y=w373) -> (x+y=w372:u32)
          }
        }
      }
    }
    "Alt Flow Starts" <- w320
    "Armed" <- w329
    "Positive Threshold" <- w328
  }
